vi "Dummy VI 4.vi"(6 "error in":errorcluster, 11 "String":string) -> (4 "error out":errorcluster)   [LabVIEW 2020]
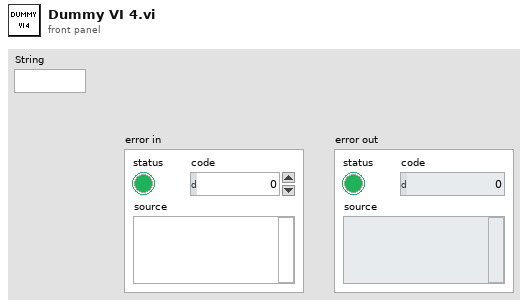
[diagram p1: front panel]
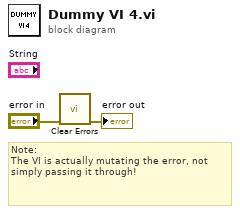
[diagram p0: block diagram]
diagram:
  # "Note:\nThe VI is actually mutating the error, not simply passing it through!"
  n1 = call <vilib>:"Clear Errors.vi"("error in (no error)"="error in") -> ("error out"=→"error out":errorcluster)  [unwired: 5 in, 1 out]
